vi "SeCrTs-Generate_Event.vi"(8 "error in":errorcluster) -> (0 "error out":errorcluster)   [LabVIEW 2022 SP3]
panel:
  in  "Output level":enum32{"low", "high"}(ring)=enum."high"
  in  "Start Time Delay (Seconds)":ext=5.0
  in  "Output Terminal":tag="/PXI1Slot4/PFI1"
  in  "resource name 2":tag="PXI1Slot4"
  out "Current time":timestamp
  out "Event Time":timestamp format="%<%I:%M:%S%9u %p\n%x>T"
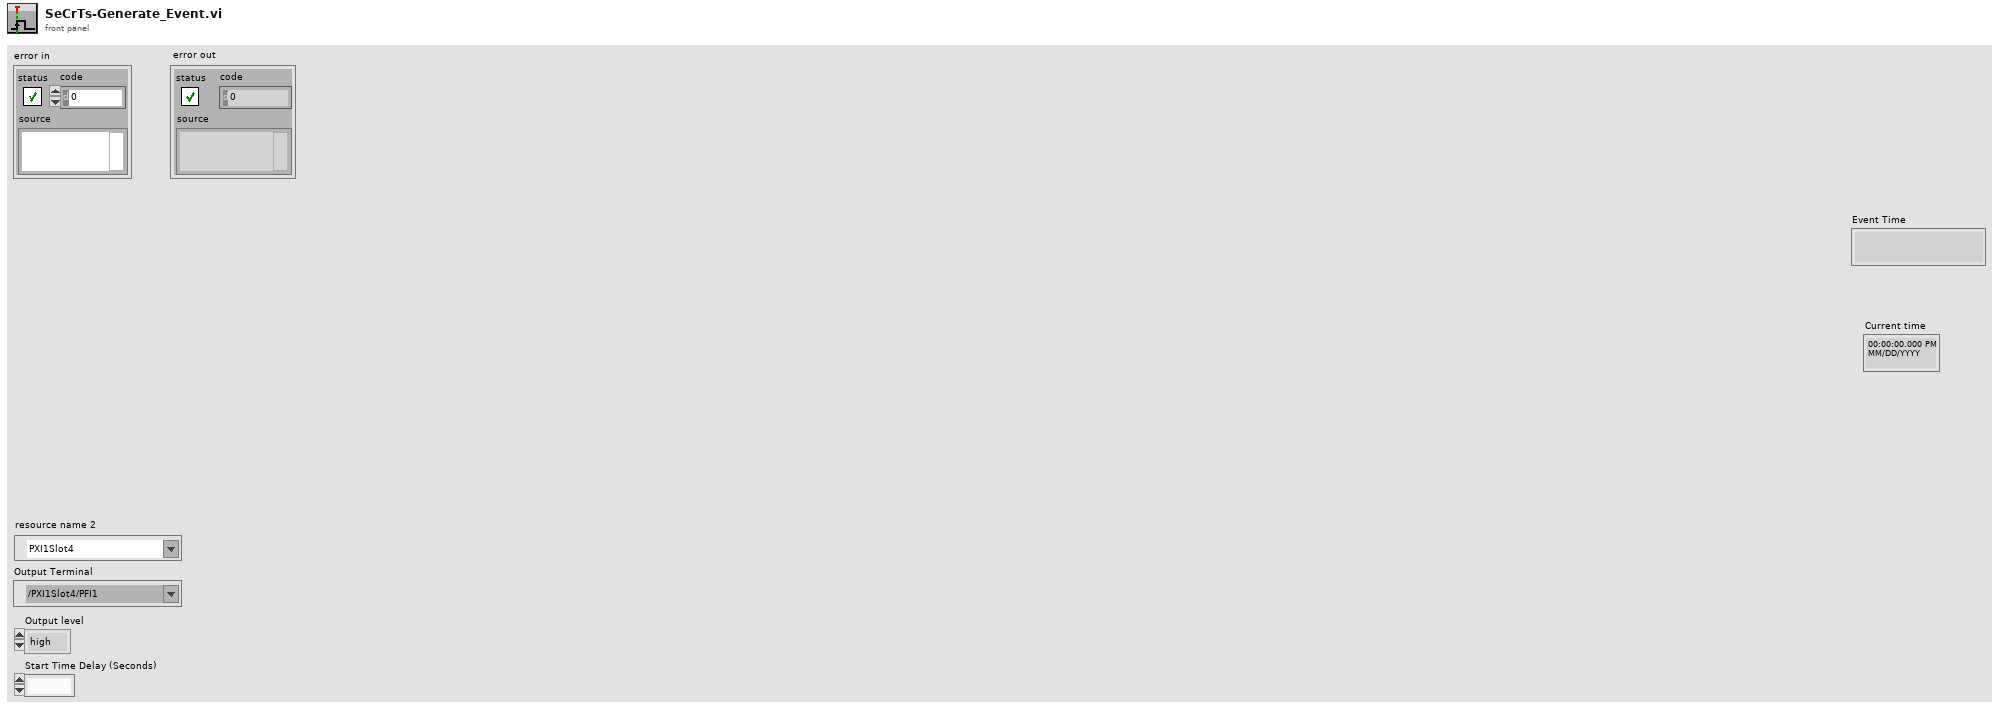
[diagram p1: front panel]
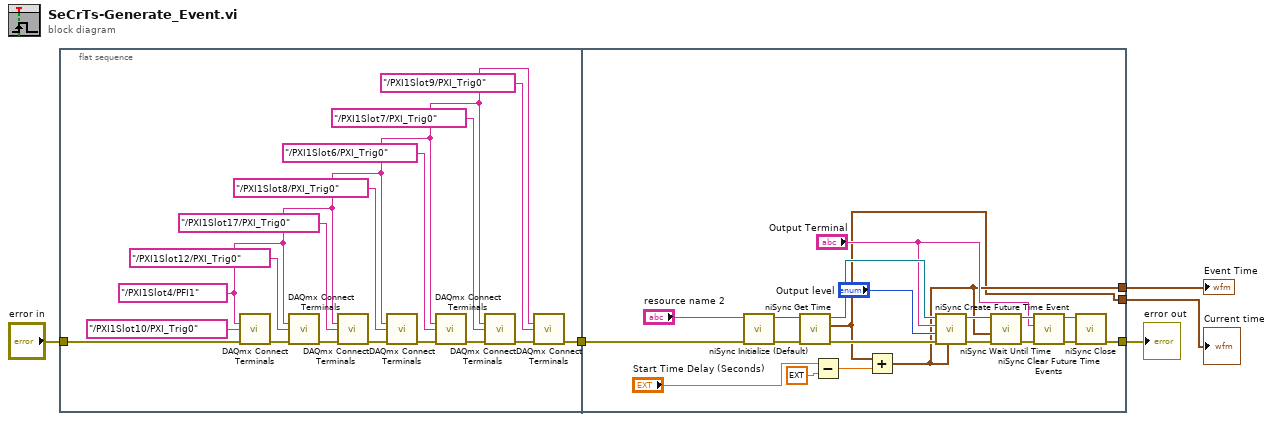
[diagram p0: block diagram]
diagram:
  n1 = flat-sequence {
    tunnel: "error in" -> [w20]
    tunnel: [w6] -> w5
    tunnel: w5 -> [w27]
    tunnel: [w24] -> w3
    tunnel: [w23] -> w2
    tunnel: [w22] -> w1
    frame #0 {
      w7 = tag "/PXI1Slot4/PFI1" ("source terminal")
      n2 = call <vilib>:"DAQmx Connect Terminals.vi"("source terminal"=w7, "destination terminal"=tag "/PXI1Slot10/PXI_Trig0", "error in"=w20) -> ("error out"=w19:errorcluster)  [unwired: 12 in]
      n3 = call <vilib>:"DAQmx Connect Terminals.vi"("source terminal"=w7, "destination terminal"=tag "/PXI1Slot12/PXI_Trig0", "error in"=w19) -> ("error out"=w17:errorcluster)  [unwired: 12 in]
      n4 = call <vilib>:"DAQmx Connect Terminals.vi"("source terminal"=w7, "destination terminal"=tag "/PXI1Slot17/PXI_Trig0", "error in"=w17) -> ("error out"=w15:errorcluster)  [unwired: 12 in]
      n5 = call <vilib>:"DAQmx Connect Terminals.vi"("source terminal"=w7, "destination terminal"=tag "/PXI1Slot8/PXI_Trig0" ("source terminal"), "error in"=w15) -> ("error out"=w13:errorcluster)  [unwired: 12 in]
      n6 = call <vilib>:"DAQmx Connect Terminals.vi"("source terminal"=w7, "destination terminal"=tag "/PXI1Slot6/PXI_Trig0", "error in"=w13) -> ("error out"=w11:errorcluster)  [unwired: 12 in]
      n7 = call <vilib>:"DAQmx Connect Terminals.vi"("source terminal"=w7, "destination terminal"=tag "/PXI1Slot7/PXI_Trig0", "error in"=w11) -> ("error out"=w9:errorcluster)  [unwired: 12 in]
      n8 = call <vilib>:"DAQmx Connect Terminals.vi"("source terminal"=w7, "destination terminal"=tag "/PXI1Slot9/PXI_Trig0", "error in"=w9) -> ("error out"=w6:errorcluster)  [unwired: 12 in]
    }
    frame #1 {
      n9 = call <instrlib>:"niSync Initialize (Default).vi"("error in (no error)"=w27, "resource name"="resource name 2") -> ("error out"=w32:errorcluster, "instrument handle out"=w33:refnum<k15>)  [unwired: 8 in]
      n10 = call <instrlib>:"niSync Get Time.vi"("error in (no error)"=w32, "instrument handle"=w33) -> ("error out"=w38:errorcluster, "time"=w23:timestamp, "instrument handle out"=w39:refnum<k15>)  [unwired: 5 in]
      n11 = Subtract(x="Start Time Delay (Seconds)", y=ext 0.2) -> (x-y=w26:ext)
      n12 = Add(x=w23, y=w26) -> (x+y=w24:timestamp)
      n13 = call <instrlib>:"niSync Create Future Time Event.vi"("time"=w24, "error in (no error)"=w38, "output level"="Output level", "terminal"="Output Terminal", "instrument handle"=w39) -> ("error out"=w36:errorcluster, "instrument handle out"=w37:refnum<k15>)  [unwired: 4 in]
      n14 = call <instrlib>:"niSync Wait Until Time.vi"("error in (no error)"=w36, "time stamp"=w24, "instrument handle"=w37) -> ("error out"=w35:errorcluster, "instrument handle out"=w34:refnum<k15>)  [unwired: 3 in]
      n15 = call <instrlib>:"niSync Clear Future Time Events.vi"("error in (no error)"=w35, "terminal"="Output Terminal", "instrument handle"=w34) -> ("error out"=w30:errorcluster, "instrument handle out"=w31:refnum<k15>)  [unwired: 6 in]
      n16 = call <instrlib>:"niSync Close.vi"("error in (no error)"=w30, "instrument handle"=w31) -> ("error out"=w22:errorcluster)  [unwired: 9 in]
    }
  }
  "error out" <- w1
  "Event Time" <- w3
  "Current time" <- w2
